vi "process_img.vi"(7 "ROI":T2, 8 "error in (no error)":errorcluster, 10 "Options":T3, 11 "Image Src":T1) -> (0 "error out":errorcluster, 3 "Image Dst":T1)   [LabVIEW 2020]
uses:
  #typedefs/#typedef_cluster_ANALYZE_Options.ctl
  <vilib>/vision/Image Controls.llb/IMAQ Image.ctl
  <vilib>/vision/NI_Vision_Development_Module.lvlib
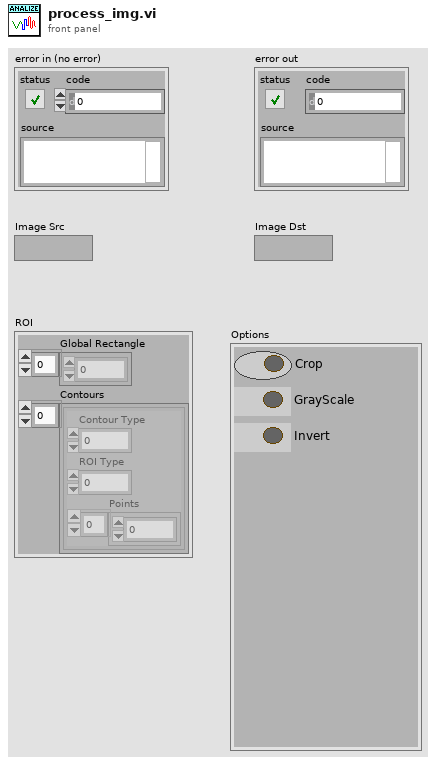
[diagram p1: front panel]
types:
  T1 = typedef "IMAQ Image.ctl" = refnum<image>
  T2 = cluster{"Global Rectangle":i32[], "Contours":cluster{"Contour Type":u32, "ROI Type":u32, "Points":i32[]}[]}
  T3 = typedef "#typedef_cluster_ANALYZE_Options.ctl" = cluster{"Crop":bool, "GrayScale":bool, "Invert":bool}
  T4 = typedef "Image Type" = u32
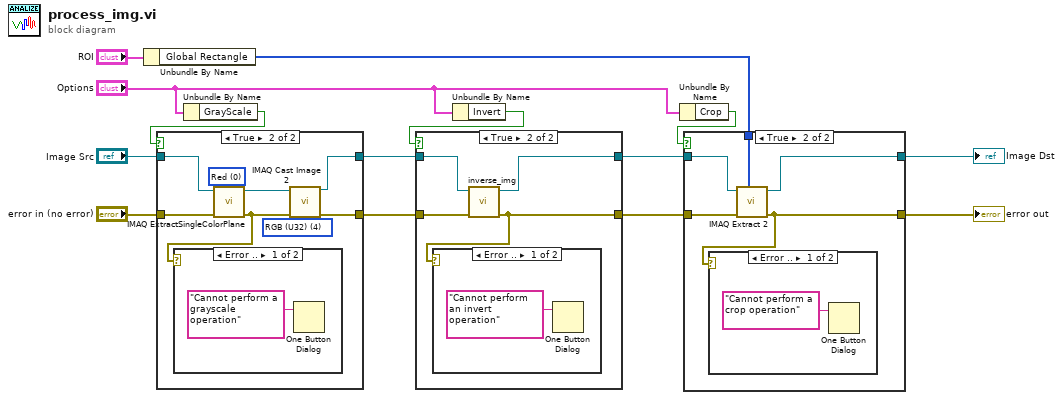
[diagram p0: block diagram]
diagram:
  n1 = Unbundle By Name("ROI") -> ("Global Rectangle"=w11:i32[])
  n2 = Unbundle By Name("Options") -> ("GrayScale"=w8:bool)
  n3 = case shown="True" w8 {
    tunnel: "error in (no error)" -> [w15 w23]
    tunnel: "Image Src" -> [w16 w22]
    tunnel: [w15 w19] -> w4
    tunnel: [w16 w17] -> w5
    frame False {
    }
    frame True {
      w18 = T4 4 items=["Grayscale (U8)", "Grayscale (I16)", "Grayscale (SGL)", "Complex (CSG)", "RGB (U32)", "HSL (U32)", "RGB (U64)", "Grayscale (U16)"] ("Image Type")
      w24 = 0 items=["Red", "Green", "Blue", "Hue", "Saturation", "Luminance", "Value", "Intensity"] ("Color Plane")
      n4 = call "IMAQ ExtractSingleColorPlane"("Color Plane"=w24, "error in (no error)"=w23, "Image Src"=w22) -> ("error out"=w20:errorcluster, "Image Dst Out"=w21:T1)  [unwired: 7 in]
      n5 = case shown="Error .." w20 {
        frame Error {
          n6 = One Button Dialog(message="Cannot perform a grayscale operation") -> ()  [unwired: 1 in, 1 out]
        }
        frame No Error {
        }
      }
      n7 = call "IMAQ Cast Image 2"("Image Src"=w21, "Image Type"=w18, "error in (no error)"=w20) -> ("Image Dst Out"=w17:T1, "error out"=w19:errorcluster)  [unwired: 11 in]
    }
  }
  n8 = Unbundle By Name("Options") -> ("Invert"=w6:bool)
  n9 = case shown="True" w6 {
    tunnel: w4 -> [w26 w31]
    tunnel: w5 -> [w27 w29]
    tunnel: [w26 w30] -> w1
    tunnel: [w27 w28] -> w2
    frame False {
    }
    frame True {
      n10 = call "inverse_img.vi"("error in (no error)"=w31, "Image Src"=w29) -> ("error out"=w30:errorcluster, "Image Dst"=w28:T1)  [unwired: 8 in]
      n11 = case shown="Error .." w30 {
        frame Error {
          n12 = One Button Dialog(message="Cannot perform an invert operation") -> ()  [unwired: 1 in, 1 out]
        }
        frame No Error {
        }
      }
    }
  }
  n13 = Unbundle By Name("Options") -> ("Crop"=w7:bool)
  n14 = case shown="True" w7 {
    tunnel: w11 -> [_ w39]
    tunnel: w1 -> [w33 w38]
    tunnel: [w33 w35] -> w10
    tunnel: w2 -> [w34 w37]
    tunnel: [w34 w36] -> w9
    frame False {
    }
    frame True {
      n15 = call "IMAQ Extract 2"("Optional Rectangle"=w39, "error in (no error)"=w38, "Image Src"=w37) -> ("error out"=w35:errorcluster, "Image Dst Out"=w36:T1)  [unwired: 7 in]
      n16 = case shown="Error .." w35 {
        frame Error {
          n17 = One Button Dialog(message="Cannot perform a crop operation") -> ()  [unwired: 1 in, 1 out]
        }
        frame No Error {
        }
      }
    }
  }
  "error out" <- w10
  "Image Dst" <- w9
